vi "Load Play.vi"(4 "Load Play":bool, 5 "Filepath Array":string[](array[string]), 6 "Play Selector Box":string, 7 "Play Currently Open Property Reference":refnum<vi>, 8 "Empty Play Definition":T1, 9 "filename array":string[](array[string]), 10 "Previous Iteration \nFile Refnum":refnum<file>, 11 "Current File Refnum":refnum<vi>) -> (0 "Read file error":errorcluster, 3 "Output File Refnum":refnum<file>)   [LabVIEW 2014]
uses:
  Autonomous VIs/Autonomous Exec/Autonomous Play Definition.ctl
  Autonomous VIs/Autonomous Commands/Autonomous Command Names.ctl
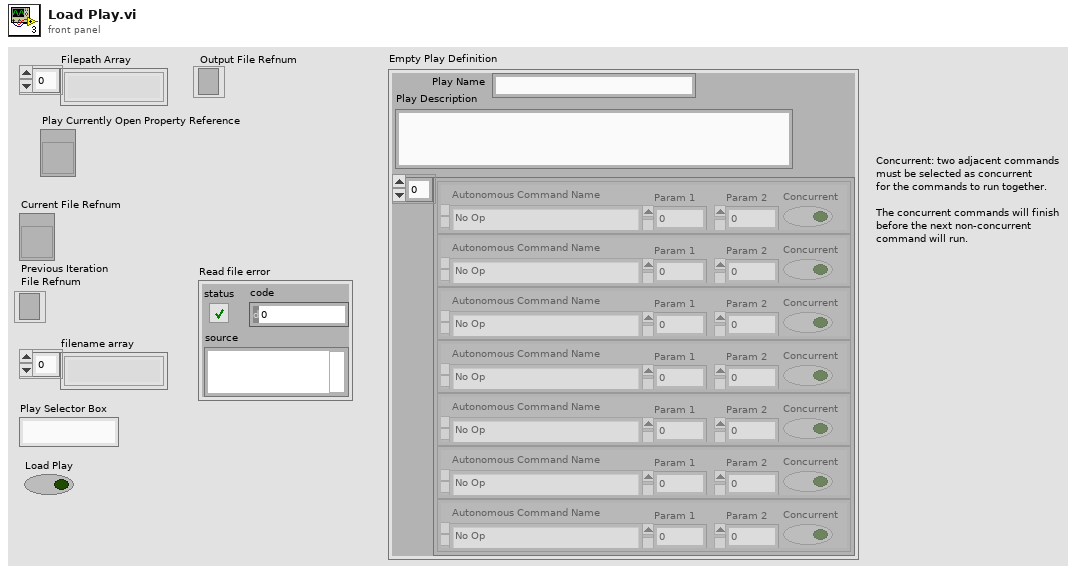
[diagram p1: front panel]
types:
  T1 = typedef "Autonomous Play Definition.ctl" = cluster{"Play Name":string, "Command List":cluster{"Param 1":dbl, "Param 2":dbl, "Autonomous Command Name":T2, "Concurrent":bool}[], "Play Description":string}
  T2 = typedef "Autonomous Command Names.ctl" = enum16{"No Op", "Drive Distance Robot", "Drive Time Robot", "Translate Distance Robot", "Translate Time Robot", "Drive Distance Field", "Drive Time Field", "Translate Distance Field", "Translate Time Field", "Rotate Robot", "Set Initial Gyro Value", "Lifter to Setpoint", "Wait", "Do Not use", "Drive Distance Field (Gyro Hold)", "Translate Distance Field (Gyro Hold)", "Can", "Grabber", "Drive Distance Field (Sensor Stop, Gyro Hold)", "Move Direction Field (Gyro Hold)", "Rotate Robot 90 about Tote", "Reset Gyro", "Find Tote", "Get Tote Into Robot", "Lower Can Grabber"}
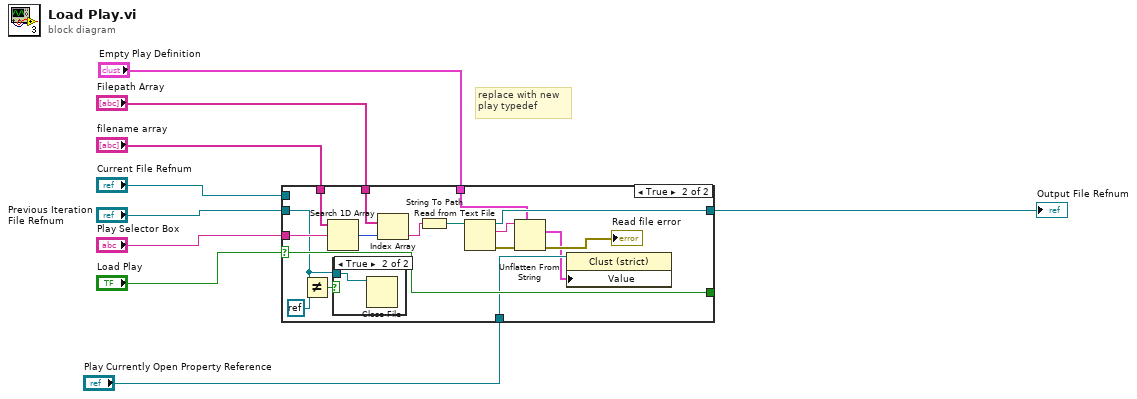
[diagram p0: block diagram]
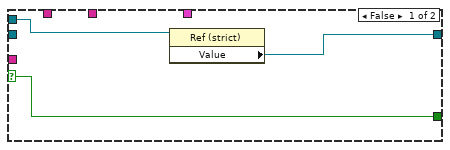
[diagram p2: hidden frame]
diagram:
  # "replace with new \nplay typedef"
  n1 = case shown="True" "Load Play" {
    selector: "Load Play" -> [w12 w21]
    tunnel: "Play Selector Box" -> [_ w25]
    tunnel: [w11 w26] -> w6
    tunnel: "Previous Iteration \nFile Refnum" -> [_ w19]
    tunnel: "filename array" -> [_ w24]
    tunnel: "Filepath Array" -> [_ w23]
    tunnel: [w12 w21] -> _
    tunnel: "Current File Refnum" -> [w10 _]
    tunnel: "Empty Play Definition" -> [_ w15]
    tunnel: "Play Currently Open Property Reference" -> [_ w14]
    frame False {
      n2 = property class="Ref (strict)"(reference=w10) -> ("Value"=w11:refnum<file>)  [unwired: 1 in, 2 out]
    }
    frame True {
      n3 = Not Equal?(x=w19, y=refnum<k0> refnum) -> (x != y?=w20:bool)
      n4 = Search 1D Array(1D array=w24, element=w25) -> (index of element=w28:i32)  [unwired: 1 in]
      n5 = case shown="True" w20 {
        tunnel: w19 -> [_ w30]
        frame False {
        }
        frame True {
          n6 = Close File(refnum=w30) -> ()  [unwired: 1 in, 2 out]
        }
      }
      n7 = Index Array(array=w23, index=w28) -> (element=w22:string)
      n8 = String To Path(string=w22) -> (path=w27:path)
      n9 = Read from Text File(file (use dialog)=w27) -> (refnum out=w26:refnum<file>, text=w29:string, error out=w16:errorcluster)  [unwired: 3 in, 1 out]
      n10 = Unflatten From String(type=w15, binary string=w29, error in (no error)=w16) -> (value=w13:T1, error out=→"Read file error":errorcluster)  [unwired: 2 in, 1 out]
      n11 = property class="Clust (strict)"(reference=w14, "Value"=w13) -> ()  [unwired: 1 in, 2 out]
    }
  }
  "Output File Refnum" <- w6
